vi "ukol1.vi"() -> ()   [LabVIEW 2022 SP3]
panel:
  in  "stop":bool
  out "Soucet 2":u32
  out "Soucet":dbl
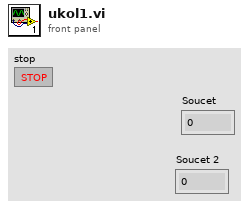
[diagram p1: front panel]
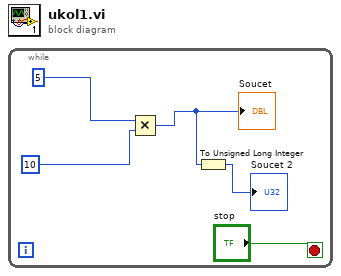
[diagram p0: block diagram]
diagram:
  n1 = while {
    stop <- "stop" stop-if-true
    n2 = Multiply(x=u32 5 ("Cislo 1"), y=u32 10 ("Cislo 2")) -> (x*y=w3:u32)
    "Soucet" <- w3
    n3 = To Unsigned Long Integer(number=w3) -> (unsigned 32bit integer=→"Soucet 2":u32)
  }
